vi "DHE_ChkAbsTime.vi"(10 "abstime":string) -> (2 "ok":bool)   [LabVIEW 2016]
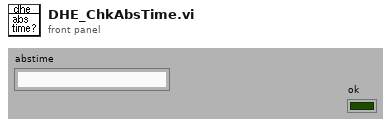
[diagram p1: front panel]
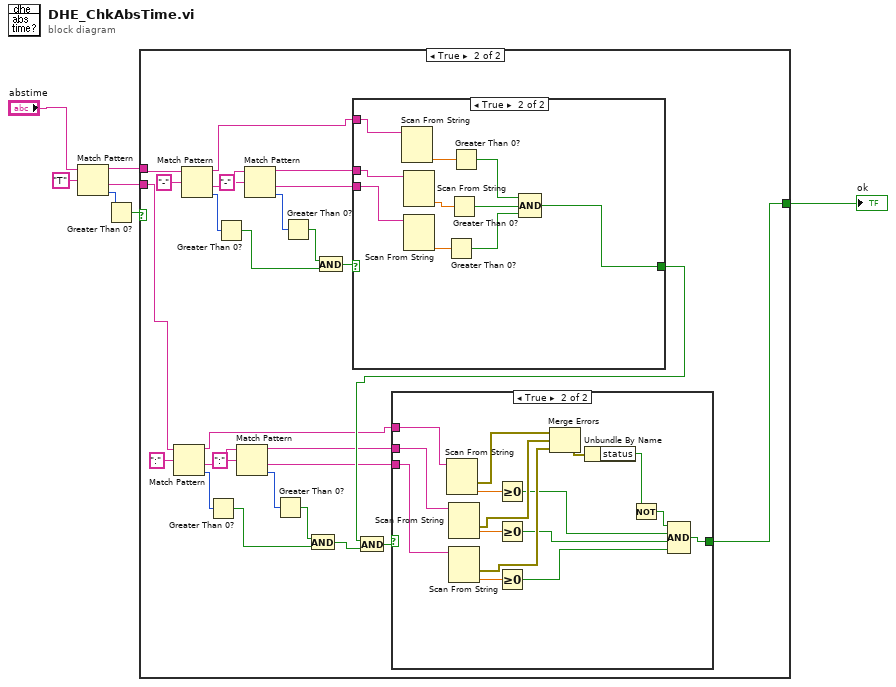
[diagram p0: block diagram]
diagram:
  n1 = Match Pattern(string="abstime", regular expression="T") -> (before substring=w2:string, after substring=w1:string, offset past match=w5:i32)  [unwired: 2 out]
  n2 = Greater Than 0?(x=w5) -> (x > 0?=w4:bool)
  n3 = case shown="True" w4 {
    selector: w4 -> [w8 _]
    tunnel: [w8 w12] -> w3
    tunnel: w2 -> [_ w35]
    tunnel: w1 -> [_ w19]
    frame False {
    }
    frame True {
      n4 = Match Pattern(string=w19, regular expression=":") -> (before substring=w11:string, after substring=w25:string, offset past match=w23:i32)  [unwired: 2 out]
      n5 = Match Pattern(string=w35, regular expression="-") -> (before substring=w18:string, after substring=w33:string, offset past match=w31:i32)  [unwired: 2 out]
      n6 = Greater Than 0?(x=w23) -> (x > 0?=w20:bool)
      n7 = Greater Than 0?(x=w31) -> (x > 0?=w28:bool)
      n8 = Match Pattern(string=w25, regular expression=":") -> (before substring=w10:string, after substring=w9:string, offset past match=w22:i32)  [unwired: 2 out]
      n9 = Match Pattern(string=w33, regular expression="-") -> (before substring=w17:string, after substring=w16:string, offset past match=w30:i32)  [unwired: 2 out]
      n10 = Greater Than 0?(x=w22) -> (x > 0?=w21:bool)
      n11 = Greater Than 0?(x=w30) -> (x > 0?=w29:bool)
      n12 = And(x=w21, y=w20) -> (x .and. y?=w14:bool)
      n13 = And(x=w29, y=w28) -> (x .and. y?=w27:bool)
      n14 = case shown="True" w27 {
        selector: w27 -> [w53 _]
        tunnel: w18 -> [_ w63]
        tunnel: w17 -> [_ w62]
        tunnel: w16 -> [_ w61]
        tunnel: [w53 w54] -> w13
        frame False {
        }
        frame True {
          n15 = Scan From String(input string=w63) -> (output 1=w60:dbl)  [unwired: 3 in, 4 out]
          n16 = Scan From String(input string=w62) -> (output 1=w58:dbl)  [unwired: 3 in, 4 out]
          n17 = Scan From String(input string=w61) -> (output 1=w57:dbl)  [unwired: 3 in, 4 out]
          n18 = Greater Than 0?(x=w57) -> (x > 0?=w55:bool)
          n19 = Greater Than 0?(x=w58) -> (x > 0?=w56:bool)
          n20 = Greater Than 0?(x=w60) -> (x > 0?=w59:bool)
          n21 = Compound Arithmetic op=AND(w59, w56, w55) -> (w54:bool)
        }
      }
      n22 = And(x=w13, y=w14) -> (x .and. y?=w15:bool)
      n23 = case shown="True" w15 {
        selector: w15 -> [w36 _]
        tunnel: [w36 w37] -> w12
        tunnel: w11 -> [_ w52]
        tunnel: w10 -> [_ w51]
        tunnel: w9 -> [_ w50]
        frame False {
        }
        frame True {
          n24 = Scan From String(input string=w52) -> (error out=w46:errorcluster, output 1=w49:dbl)  [unwired: 3 in, 3 out]
          n25 = Scan From String(input string=w51) -> (error out=w45:errorcluster, output 1=w47:dbl)  [unwired: 3 in, 3 out]
          n26 = Scan From String(input string=w50) -> (error out=w44:errorcluster, output 1=w48:dbl)  [unwired: 3 in, 3 out]
          n27 = Greater Or Equal To 0?(x=w49) -> (x >= 0?=w43:bool)
          n28 = Greater Or Equal To 0?(x=w47) -> (x >= 0?=w42:bool)
          n29 = Greater Or Equal To 0?(x=w48) -> (x >= 0?=w41:bool)
          n30 = Merge Errors(w46, w45, w44) -> (w40:errorcluster)
          n31 = Unbundle By Name(w40) -> ("status"=w39:bool)
          n32 = Not(x=w39) -> (.not. x?=w38:bool)
          n33 = Compound Arithmetic op=AND(w38, w43, w42, w41) -> (w37:bool)
        }
      }
    }
  }
  "ok" <- w3
